vi "Read All source names.vi"(11 "SolutionBuilder in":refnum<class "SolutionBuilder.lvclass">) -> (2 "All source names":set{string}(c389), 3 "SolutionBuilder out":refnum<class "SolutionBuilder.lvclass">)   [LabVIEW 2020, in "SolutionBuilder.lvlib" / "SolutionBuilder.lvclass"]
uses:
  SolutionBuilder.lvclass
  ProjectItem/ProjectItem.lvclass
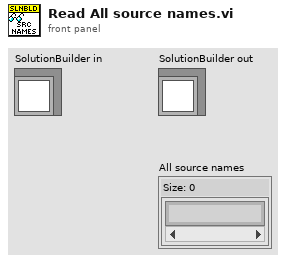
[diagram p1: front panel]
types:
  T1 = typedef "SolutionBuilder.lvlib/SolutionBuilder.lvclass/ProjectItemMap.ctl" = map{path, refnum<class "ProjectItem.lvclass">[]}
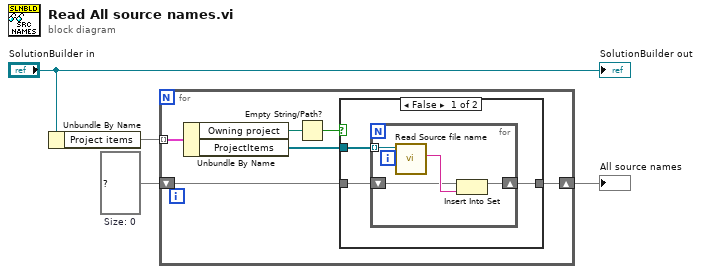
[diagram p0: block diagram]
diagram:
  w2 = set{string} {}  # Size: 0
  n1 = Unbundle By Name("SolutionBuilder in") -> ("Project items"=w3:T1)
  n2 = for {
    tunnel: w3 -> [w10] mode=indexing
    shift-right: [w6] -> w1
    shift-left: w2 -> [w5]
    n3 = Unbundle By Name(w10) -> ("Owning project"=w9:path, "ProjectItems"=w7:refnum<class "ProjectItem.lvclass">[])
    n4 = Empty String/Path?(string/path=w9) -> (empty?=w8:bool)
    n5 = case shown="False" w8 {
      tunnel: w7 -> [w13 _]
      tunnel: [w12 w18] -> w6
      tunnel: w5 -> [w11 w18]
      frame False {
        n6 = for {
          tunnel: w13 -> [w17] mode=indexing
          shift-right: [w15] -> w12
          shift-left: w11 -> [w14]
          n7 = call-dynamic "Read Source file name.vi"("ProjectItem in"=w17) -> ("Source file name"=w16:string)  [unwired: 9 in, 1 out]
          n8 = Insert Into Set(10:w16, 11:w14) -> (3:w15:set{string})  [unwired: 1 out]
        }
      }
      frame True {
      }
    }
  }
  "All source names" <- w1
  "SolutionBuilder out" <- "SolutionBuilder in"
